vi "Execute.vi"(8 "error in":errorcluster, 11 "Speaker STEP in":refnum<class "Speaker STEP.lvclass">) -> (0 "error out":errorcluster, 1 "Next Step?":bool, 2 "MSG":string, 3 "Speaker STEP out":refnum<class "Speaker STEP.lvclass">)   [LabVIEW 2014, in "Speaker STEP.lvclass"]
uses:
  Speaker STEP.lvclass
  <vilib>/ActorFramework/Message Enqueuer/Message Enqueuer.lvclass
  Controller/Messages/Change Speaker MSG/Speaker MSG.lvclass
  reusable/Sequence/STEPS/STEP.lvclass/STEP.ctl
  Controller/Messages/Change Speaker MSG/Speaker MSG.lvclass/Speaker MSG.ctl
  <vilib>/ActorFramework/Message Enqueuer/Message Enqueuer.lvclass/Message Enqueuer.ctl
  reusable/Sequence/STEPS/Read Obj.vi
  Controller/Messages/Change Speaker MSG/Write spk.vi
  <vilib>/ActorFramework/Message Priority Queue/Priority Enqueue.vi
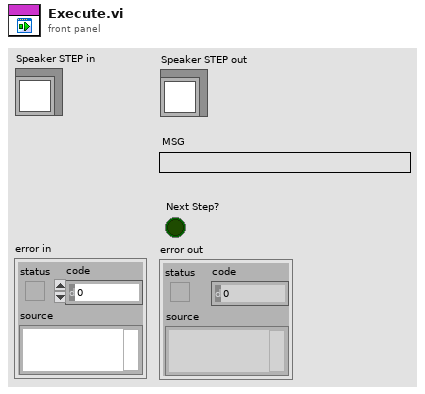
[diagram p1: front panel]
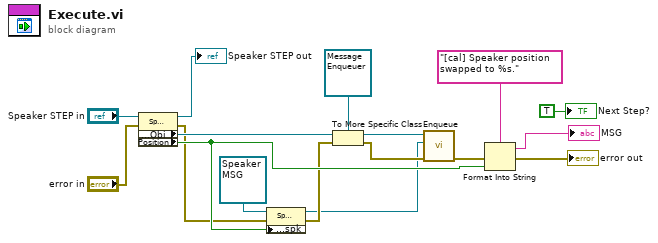
[diagram p0: block diagram]
diagram:
  n1 = property class="Speaker"(reference="Speaker STEP in", error in="error in") -> (reference out=→"Speaker STEP out":refnum<class "Speaker STEP.lvclass">, error out=w3:errorcluster, "Accessors:Obj"=w17:refnum<class>, "Position"=w4:bool)
  n2 = property class="Speaker MSG.lvclass"(reference=refnum<class "Speaker MSG.lvclass"> refnum ("Controller:Speaker MSG.lvclass"), error in=w3, "Accessors:spk"=w4) -> (reference out=w1:refnum<class "Speaker MSG.lvclass">, error out=w2:errorcluster)
  n3 = To More Specific Class(target class=refnum<class "Message Enqueuer.lvclass"> refnum ("Message Enqueuer in"), reference=w17, error in=w2) -> (specific class reference=w14:refnum<class "Message Enqueuer.lvclass">, error out=w15:errorcluster)
  n4 = call <vilib>:"Enqueue.vi"("error in (no error)"=w15, "Message"=w1, "Message Enqueuer in"=w14) -> ("error out"=w12:errorcluster)  [unwired: 7 in, 1 out]
  n5 = Format Into String(format string="[cal] Speaker position swapped to %s.", error in=w12, w4) -> (resulting string=→"MSG":string, error out=→"error out":errorcluster)  [unwired: 1 in]
  "Next Step?" <- TRUE
